vi "FRIC_navX_Get_Status.vi"(5 "Device Number":T1, 7 "Update":bool) -> (2 "Status":T4 {"OP Status" items=["INITIALIZING", "SELFTEST_IN_PROGRESS", "ERROR", "IMU_AUTOCAL_IN_PROGRESS", "NORMAL"]; "Calibration Status" items=["IMU_CAL_STATE_MASK"=3, "IMU_CAL_STATE_INPROGRESS"=0, "IMU_CAL_STATE_ACCUMULATE"=1, "IMU_CAL_STATE_COMPLETE"=2]})   [LabVIEW 2016]
doc: "This navX VI returns the current status of the navX."
uses:
  _TypeDefs/Flags/Z900_navX_Flags_OpStatusTypeDef.ctl
  _TypeDefs/Flags/Z900_navX_Flags_CalibrationStatusTypeDef.ctl
  _TypeDefs/FRIC_navX_DeviceNumbersTypeDef.ctl
  _TypeDefs/Z900_navX_DeviceRegisters.ctl
  _TypeDefs/Flags/Z900_navX_Flags_SelfTestStatusTypeDef.ctl
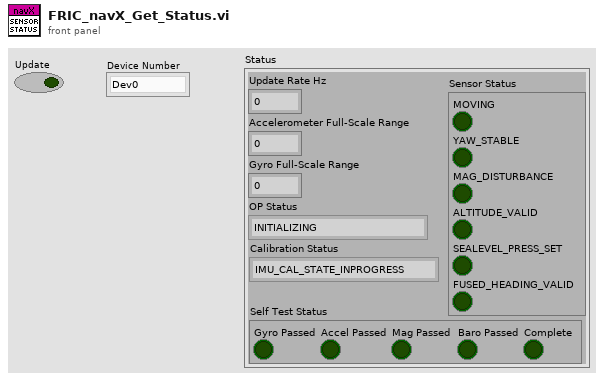
[diagram p1: front panel]
types:
  T1 = typedef "FRIC_navX_DeviceNumbersTypeDef.ctl" = enum16{"Dev0", "Dev1", "Dev2", "Dev3", "Dev4", "Dev5", "Dev6", "Dev7", "Dev8", "Dev9", "Dev10"}
  T2 = typedef "Z900_navX_Flags_OpStatusTypeDef.ctl" = u8
  T3 = typedef "Z900_navX_Flags_CalibrationStatusTypeDef.ctl" = u8
  T4 = cluster{"Update Rate Hz":u8, "Accelerometer Full-Scale Range":u8, "Gyro Full-Scale Range":u16, "OP Status":T2, "Calibration Status":T3, "Sensor Status":cluster{"MOVING":bool, "YAW_STABLE":bool, "MAG_DISTURBANCE":bool, "ALTITUDE_VALID":bool, "SEALEVEL_PRESS_SET":bool, "FUSED_HEADING_VALID":bool}, "Self Test Status":cluster{"Gyro Passed":bool, "Accel Passed":bool, "Mag Passed":bool, "Baro Passed":bool, "Complete":bool}}
  T5 = cluster{"MOVING":bool, "YAW_STABLE":bool, "MAG_DISTURBANCE":bool, "ALTITUDE_VALID":bool, "SEALEVEL_PRESS_SET":bool, "FUSED_HEADING_VALID":bool}
  T6 = cluster{"Gyro Passed":bool, "Accel Passed":bool, "Mag Passed":bool, "Baro Passed":bool, "Complete":bool}
  T7 = typedef "Z900_navX_Flags_SelfTestStatusTypeDef.ctl" = u8
  T8 = typedef "Z900_navX_DeviceRegisters.ctl" = u8
  T9 = cluster{"Update Rate Hz":u8, "Accelerometer Full-Scale Range":u8, "Gyro Full-Scale Range":u16, "OP Status":T2, "Calibration Status":T3, "Sensor Status":cluster{"MOVING":bool, "YAW_STABLE":bool, "MAG_DISTURBANCE":bool, "ALTITUDE_VALID":bool, "SEALEVEL_PRESS_SET":bool, "FUSED_HEADING_VALID":bool}, "Self Test Status":cluster{"Gyro Passed":bool, "Accel Passed":bool, "Mag Passed":bool, "Baro Passed":bool, "Complete":bool}}[]
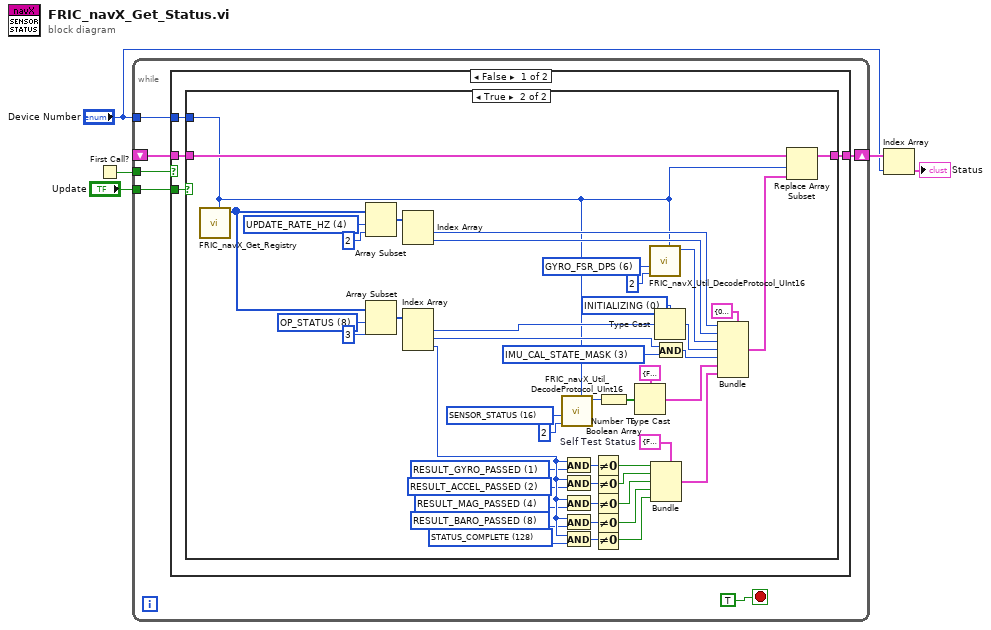
[diagram p0: block diagram]
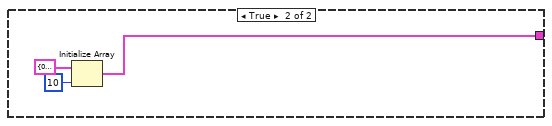
[diagram p3: hidden frame]
diagram:
  n1 = First Call?() -> (First Call?: T/F=w4:bool)
  n2 = while {
    shift-right: [w11] -> w3
    shift-left: _ -> [w8]
    tunnel: "Update" -> [w9]
    tunnel: "Device Number" -> [w7]
    tunnel: w4 -> [w6]
    stop <- TRUE stop-if-true
    n3 = case shown="False" w6 {
      tunnel: [w15 w64] -> w11
      tunnel: w9 -> [w14 _]
      tunnel: w8 -> [w13 _]
      tunnel: w7 -> [w12 _]
      frame False {
        n4 = case shown="True" w14 {
          tunnel: [w16 w19] -> w15
          tunnel: w13 -> [w16 w20]
          tunnel: w12 -> [_ w17]
          frame False {
          }
          frame True {
            w21 = T6 {"Gyro Passed"=FALSE, "Accel Passed"=FALSE, "Mag Passed"=FALSE, "Baro Passed"=FALSE, "Complete"=FALSE}  # Self Test Status
            w28 = T7 128 items=["STATUS_COMPLETE"=128, "RESULT_GYRO_PASSED"=1, "RESULT_ACCEL_PASSED"=2, "RESULT_MAG_PASSED"=4, "RESULT_BARO_PASSED"=8] ("Self Test Status")
            w29 = T7 8 items=["STATUS_COMPLETE"=128, "RESULT_GYRO_PASSED"=1, "RESULT_ACCEL_PASSED"=2, "RESULT_MAG_PASSED"=4, "RESULT_BARO_PASSED"=8] ("Self Test Status")
            w32 = T7 4 items=["STATUS_COMPLETE"=128, "RESULT_GYRO_PASSED"=1, "RESULT_ACCEL_PASSED"=2, "RESULT_MAG_PASSED"=4, "RESULT_BARO_PASSED"=8] ("Self Test Status")
            w33 = T7 2 items=["STATUS_COMPLETE"=128, "RESULT_GYRO_PASSED"=1, "RESULT_ACCEL_PASSED"=2, "RESULT_MAG_PASSED"=4, "RESULT_BARO_PASSED"=8] ("Self Test Status")
            w36 = T7 1 items=["STATUS_COMPLETE"=128, "RESULT_GYRO_PASSED"=1, "RESULT_ACCEL_PASSED"=2, "RESULT_MAG_PASSED"=4, "RESULT_BARO_PASSED"=8] ("Self Test Status")
            w38 = T8 8 items=["WHOAMI"=0, "HW_REV"=1, "FW_VER_MAJOR"=2, "FW_VER_MINOR"=3, "UPDATE_RATE_HZ"=4, "ACCEL_FSR_G"=5, "GYRO_FSR_DPS"=6, "OP_STATUS"=8, "CAL_STATUS"=9, "SELFTEST_STATUS"=10, "CAPABILITY_FLAGS_L"=11, "CAPABILITY_FLAGS_H"=12, "SENSOR_STATUS"=16, "TIMESTAMP"=18, "YAW"=22, "ROLL"=24, "PITCH"=26, "HEADING"=28, "FUSED_HEADING"=30, "ALTITUDE_I"=32, "ALTITUDE_D"=34, "LINERA_ACC_X"=36, "LINERA_ACC_Y"=38, "LINERA_ACC_Z"=40, "QUAT_W"=42, "QUAT_X"=44, "QUAT_Y"=46, "QUAT_Z"=48, "MPU_TEMP_C"=50, "GYRO_X"=52, "GYRO_Y"=54, "GYRO_Z"=56, "ACC_X"=58, "ACC_Y"=60, "ACC_Z"=62, "MAG_X"=64, "MAG_Y"=66, "MAG_Z"=68, "PRESSURE_I"=70, "PRESSURE_D"=72, "PRESSURE_TEMP"=74, "YAW_OFFSET"=76, "QUAT_OFFSET_W"=78, "QUAT_OFFSET_X"=80, "QUAT_OFFSET_Y"=82, "QUAT_OFFSET_Z"=84, "INTEGRATION_CONTROL"=86, "VELOCITY_X"=88, "VELOCITY_Y"=92, "VELOCITY_Z"=96, "DISPLACMENT_X"=100, "DISPLACMENT_Y"=104, "DISPLACEMENT_Z"=108] ("Device Register")
            w40 = T8 4 items=["WHOAMI"=0, "HW_REV"=1, "FW_VER_MAJOR"=2, "FW_VER_MINOR"=3, "UPDATE_RATE_HZ"=4, "ACCEL_FSR_G"=5, "GYRO_FSR_DPS"=6, "OP_STATUS"=8, "CAL_STATUS"=9, "SELFTEST_STATUS"=10, "CAPABILITY_FLAGS_L"=11, "CAPABILITY_FLAGS_H"=12, "SENSOR_STATUS"=16, "TIMESTAMP"=18, "YAW"=22, "ROLL"=24, "PITCH"=26, "HEADING"=28, "FUSED_HEADING"=30, "ALTITUDE_I"=32, "ALTITUDE_D"=34, "LINERA_ACC_X"=36, "LINERA_ACC_Y"=38, "LINERA_ACC_Z"=40, "QUAT_W"=42, "QUAT_X"=44, "QUAT_Y"=46, "QUAT_Z"=48, "MPU_TEMP_C"=50, "GYRO_X"=52, "GYRO_Y"=54, "GYRO_Z"=56, "ACC_X"=58, "ACC_Y"=60, "ACC_Z"=62, "MAG_X"=64, "MAG_Y"=66, "MAG_Z"=68, "PRESSURE_I"=70, "PRESSURE_D"=72, "PRESSURE_TEMP"=74, "YAW_OFFSET"=76, "QUAT_OFFSET_W"=78, "QUAT_OFFSET_X"=80, "QUAT_OFFSET_Y"=82, "QUAT_OFFSET_Z"=84, "INTEGRATION_CONTROL"=86, "VELOCITY_X"=88, "VELOCITY_Y"=92, "VELOCITY_Z"=96, "DISPLACMENT_X"=100, "DISPLACMENT_Y"=104, "DISPLACEMENT_Z"=108] ("Device Register")
            w44 = T8 16 items=["WHOAMI"=0, "HW_REV"=1, "FW_VER_MAJOR"=2, "FW_VER_MINOR"=3, "UPDATE_RATE_HZ"=4, "ACCEL_FSR_G"=5, "GYRO_FSR_DPS"=6, "OP_STATUS"=8, "CAL_STATUS"=9, "SELFTEST_STATUS"=10, "CAPABILITY_FLAGS_L"=11, "CAPABILITY_FLAGS_H"=12, "SENSOR_STATUS"=16, "TIMESTAMP"=18, "YAW"=22, "ROLL"=24, "PITCH"=26, "HEADING"=28, "FUSED_HEADING"=30, "ALTITUDE_I"=32, "ALTITUDE_D"=34, "LINERA_ACC_X"=36, "LINERA_ACC_Y"=38, "LINERA_ACC_Z"=40, "QUAT_W"=42, "QUAT_X"=44, "QUAT_Y"=46, "QUAT_Z"=48, "MPU_TEMP_C"=50, "GYRO_X"=52, "GYRO_Y"=54, "GYRO_Z"=56, "ACC_X"=58, "ACC_Y"=60, "ACC_Z"=62, "MAG_X"=64, "MAG_Y"=66, "MAG_Z"=68, "PRESSURE_I"=70, "PRESSURE_D"=72, "PRESSURE_TEMP"=74, "YAW_OFFSET"=76, "QUAT_OFFSET_W"=78, "QUAT_OFFSET_X"=80, "QUAT_OFFSET_Y"=82, "QUAT_OFFSET_Z"=84, "INTEGRATION_CONTROL"=86, "VELOCITY_X"=88, "VELOCITY_Y"=92, "VELOCITY_Z"=96, "DISPLACMENT_X"=100, "DISPLACMENT_Y"=104, "DISPLACEMENT_Z"=108] ("Device Register")
            w47 = T8 6 items=["WHOAMI"=0, "HW_REV"=1, "FW_VER_MAJOR"=2, "FW_VER_MINOR"=3, "UPDATE_RATE_HZ"=4, "ACCEL_FSR_G"=5, "GYRO_FSR_DPS"=6, "OP_STATUS"=8, "CAL_STATUS"=9, "SELFTEST_STATUS"=10, "CAPABILITY_FLAGS_L"=11, "CAPABILITY_FLAGS_H"=12, "SENSOR_STATUS"=16, "TIMESTAMP"=18, "YAW"=22, "ROLL"=24, "PITCH"=26, "HEADING"=28, "FUSED_HEADING"=30, "ALTITUDE_I"=32, "ALTITUDE_D"=34, "LINERA_ACC_X"=36, "LINERA_ACC_Y"=38, "LINERA_ACC_Z"=40, "QUAT_W"=42, "QUAT_X"=44, "QUAT_Y"=46, "QUAT_Z"=48, "MPU_TEMP_C"=50, "GYRO_X"=52, "GYRO_Y"=54, "GYRO_Z"=56, "ACC_X"=58, "ACC_Y"=60, "ACC_Z"=62, "MAG_X"=64, "MAG_Y"=66, "MAG_Z"=68, "PRESSURE_I"=70, "PRESSURE_D"=72, "PRESSURE_TEMP"=74, "YAW_OFFSET"=76, "QUAT_OFFSET_W"=78, "QUAT_OFFSET_X"=80, "QUAT_OFFSET_Y"=82, "QUAT_OFFSET_Z"=84, "INTEGRATION_CONTROL"=86, "VELOCITY_X"=88, "VELOCITY_Y"=92, "VELOCITY_Z"=96, "DISPLACMENT_X"=100, "DISPLACMENT_Y"=104, "DISPLACEMENT_Z"=108] ("Device Register")
            w59 = T3 3 items=["IMU_CAL_STATE_MASK"=3, "IMU_CAL_STATE_INPROGRESS"=0, "IMU_CAL_STATE_ACCUMULATE"=1, "IMU_CAL_STATE_COMPLETE"=2] ("CalibrationStatus")
            w61 = T2 0 items=["INITIALIZING", "SELFTEST_IN_PROGRESS", "ERROR", "IMU_AUTOCAL_IN_PROGRESS", "NORMAL"] ("OP Status")
            n5 = call "FRIC_navX_Get_Registry.vi"("Device Number"=w17) -> ("Registry (out)"=w37:u8[])  [unwired: 9 in, 1 out]
            n6 = Array Subset(array=w37, index=w40, length=2) -> (w53:u8[])
            n7 = Array Subset(array=w37, index=w38, length=3) -> (w63:u8[])
            n8 = Index Array(array=w53) -> (element #1=w51:u8, element #2=w52:u8)  [unwired: 2 in]
            n9 = Index Array(array=w63) -> (element #1=w62:u8, element #2=w60:u8, element #3=w50:u8)  [unwired: 3 in]
            n10 = call "FRIC_navX_Util_DecodeProtocol_UInt16.vi"("Device Number"=w17, "length"=2, "Device Register"=w44) -> ("Value"=w42:u16)  [unwired: 8 in]
            n11 = And(x=w50, y=w36) -> (x .and. y?=w35:T7)
            n12 = And(x=w50, y=w33) -> (x .and. y?=w34:T7)
            n13 = And(x=w50, y=w32) -> (x .and. y?=w31:T7)
            n14 = And(x=w50, y=w29) -> (x .and. y?=w30:T7)
            n15 = And(x=w50, y=w28) -> (x .and. y?=w27:T7)
            n16 = Not Equal To 0?(x=w35) -> (x != 0?=w26:bool)
            n17 = Not Equal To 0?(x=w34) -> (x != 0?=w25:bool)
            n18 = Not Equal To 0?(x=w31) -> (x != 0?=w24:bool)
            n19 = Not Equal To 0?(x=w30) -> (x != 0?=w23:bool)
            n20 = Not Equal To 0?(x=w27) -> (x != 0?=w22:bool)
            n21 = Number To Boolean Array(number=w42) -> (Boolean array=w55:bool[])
            n22 = Type Cast(type=T5 {"MOVING"=FALSE, "YAW_STABLE"=FALSE, "MAG_DISTURBANCE"=FALSE, "ALTITUDE_VALID"=FALSE, "SEALEVEL_PRESS_SET"=FALSE, "FUSED_HEADING_VALID"=FALSE} ("NAVX_SENSOR_STATUS"), x=w55) -> (*(type *) &x=w49:T5)
            n23 = call "FRIC_navX_Util_DecodeProtocol_UInt16.vi"("Device Number"=w17, "length"=2, "Device Register"=w47) -> ("Value"=w45:u16)  [unwired: 8 in]
            n24 = Bundle(cluster=w21, "Gyro Passed"=w26, "Accel Passed"=w25, "Mag Passed"=w24, "Baro Passed"=w23, "Complete"=w22) -> (w48:T6)
            n25 = Type Cast(type=w61, x=w62) -> (*(type *) &x=w57:T2)
            n26 = And(x=w60, y=w59) -> (x .and. y?=w56:T3)
            n27 = Bundle(cluster=T4 {"Update Rate Hz"=0, "Accelerometer Full-Scale Range"=0, "Gyro Full-Scale Range"=0, "OP Status"=0, "Calibration Status"=3, "Sensor Status"={"MOVING"=FALSE, "YAW_STABLE"=FALSE, "MAG_DISTURBANCE"=FALSE, "ALTITUDE_VALID"=FALSE, "SEALEVEL_PRESS_SET"=FALSE, "FUSED_HEADING_VALID"=FALSE}, "Self Test Status"={"Gyro Passed"=FALSE, "Accel Passed"=FALSE, "Mag Passed"=FALSE, "Baro Passed"=FALSE, "Complete"=FALSE}}, "Update Rate Hz"=w51, "Accelerometer Full-Scale Range"=w52, "Gyro Full-Scale Range"=w45, "OP Status"=w57, "Calibration Status"=w56, "Sensor Status"=w49, "Self Test Status"=w48) -> (w18:T4)
            n28 = Replace Array Subset(array=w20, new element=w18, index=w17) -> (w19:T9)
          }
        }
      }
      frame True {
        n29 = Initialize Array(T4 {"Update Rate Hz"=0, "Accelerometer Full-Scale Range"=0, "Gyro Full-Scale Range"=0, "OP Status"=0, "Calibration Status"=0, "Sensor Status"={"MOVING"=FALSE, "YAW_STABLE"=FALSE, "MAG_DISTURBANCE"=FALSE, "ALTITUDE_VALID"=FALSE, "SEALEVEL_PRESS_SET"=FALSE, "FUSED_HEADING_VALID"=FALSE}, "Self Test Status"={"Gyro Passed"=FALSE, "Accel Passed"=FALSE, "Mag Passed"=FALSE, "Baro Passed"=FALSE, "Complete"=FALSE}}, 10 ("dimension size")) -> (w64:T9)
      }
    }
  }
  n30 = Index Array(array=w3, index="Device Number") -> (element=→"Status":T4)
